vi "arduinoReadClock.vi"(8 "error in":errorcluster, 11 "Arduino Resource":T1={"VISA resource"="", "Board Type"=enum."Uno", "Connection Type"=enum."USB / Serial", "Bytes Per Packet (15)"=15}) -> (0 "error out":errorcluster, 2 "resulting string":string, 3 "Arduino Resource 2":T1={"VISA resource"="", "Board Type"=enum."Uno", "Connection Type"=enum."USB / Serial", "Bytes Per Packet (15)"=15})   [LabVIEW 2019]
uses:
  <vilib>/LabVIEW Interface for Arduino/Type Defs/Arduino Resource.ctl
  <vilib>/LabVIEW Interface for Arduino/Type Defs/Board Type.ctl
  <vilib>/LabVIEW Interface for Arduino/LabVIEW Interface for Arduino.lvlib
panel:
  out "output string":string
  out "year":u8
  out "month":u8
  out "day":u8
  out "hours":u8
  out "minutes":u8
  out "seconds":u8
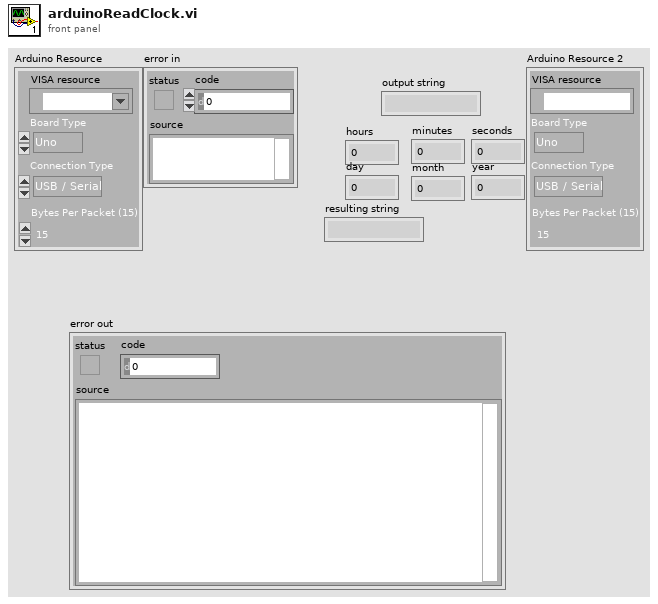
[diagram p1: front panel]
types:
  T1 = typedef "LabVIEW Interface for Arduino.lvlib/Arduino Resource.ctl" = cluster{"VISA resource":refnum<visa-resource-name>, "Board Type":T2, "Connection Type":enum8{"USB / Serial"}, "Bytes Per Packet (15)":u8}
  T2 = typedef "LabVIEW Interface for Arduino.lvlib/Board Type.ctl" = enum16{"Uno", "Dimuelanove w/Atmega 328", "Mega 2560"}
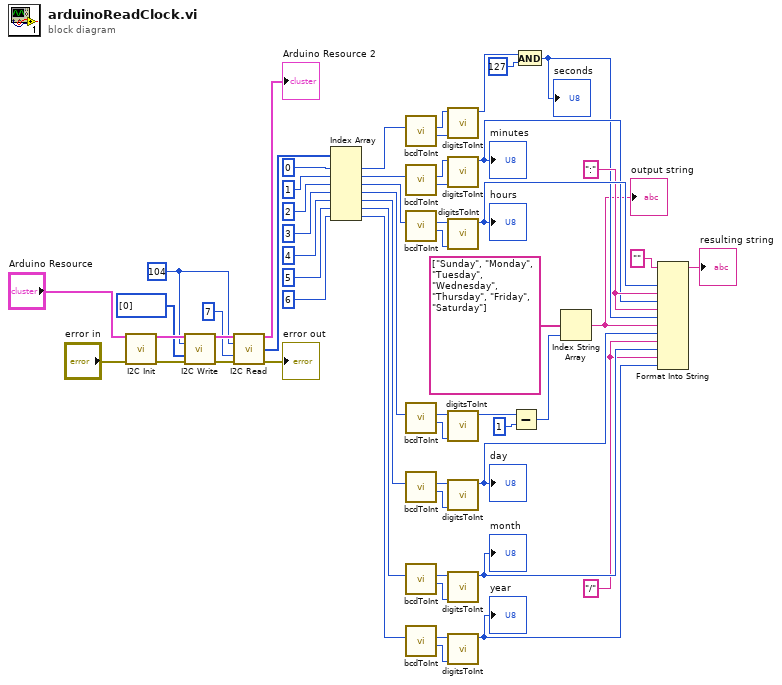
[diagram p0: block diagram]
diagram:
  w1 = "/"
  w7 = ":"
  w20 = u8 104 ("Address (0)")
  n1 = call <vilib>:"I2C Init.vi"("Arduino Resource"="Arduino Resource", "error in"="error in") -> ("Arduino Resource"=w57:T1, "error out"=w56:errorcluster)  [unwired: 12 in]
  n2 = call <vilib>:"I2C Write.vi"("Arduino Resource"=w57, "Address (0)"=w20, "I2C Data Bytes"=u8[] [0], "error in"=w56) -> ("Arduino Resource"=w54:T1, "error out"=w53:errorcluster)  [unwired: 10 in]
  n3 = call <vilib>:"I2C Read.vi"("Arduino Resource"=w54, "Address (0)"=w20, "Bytes To Read"=u8 7, "error in"=w53) -> ("Arduino Resource"=→"Arduino Resource 2":T1, "I2C Data"=w51:u8[], "error out"=→"error out":errorcluster)  [unwired: 9 in]
  n4 = Index Array(array=w51, index #1=0 ("index"), index #2=1 ("index"), index #3=2 ("index"), index #4=3 ("index"), index #5=4 ("index"), index #6=5 ("index"), index #7=6 ("index")) -> (element #1=w43:u8, element #2=w42:u8, element #3=w41:u8, element #4=w23:u8, element #5=w40:u8, element #6=w39:u8, element #7=w38:u8)
  n5 = call "bcdToInt.vi"("y"=w43) -> ("x .and. y?"=w36:u8, "x << y"=w37:u8)  [unwired: 9 in]
  n6 = call "bcdToInt.vi"("y"=w42) -> ("x .and. y?"=w27:u8, "x << y"=w26:u8)  [unwired: 9 in]
  n7 = call "bcdToInt.vi"("y"=w41) -> ("x .and. y?"=w29:u8, "x << y"=w28:u8)  [unwired: 9 in]
  n8 = call "bcdToInt.vi"("y"=w23) -> ("x .and. y?"=w25:u8, "x << y"=w24:u8)  [unwired: 9 in]
  n9 = call "bcdToInt.vi"("y"=w40) -> ("x .and. y?"=w31:u8, "x << y"=w30:u8)  [unwired: 9 in]
  n10 = call "bcdToInt.vi"("y"=w39) -> ("x .and. y?"=w33:u8, "x << y"=w32:u8)  [unwired: 9 in]
  n11 = call "bcdToInt.vi"("y"=w38) -> ("x .and. y?"=w34:u8, "x << y"=w35:u8)  [unwired: 9 in]
  n12 = call "digitsToInt.vi"("Numeric"=w36, "Numeric 2"=w37) -> ("x+y"=w22:u8)  [unwired: 9 in]
  n13 = call "digitsToInt.vi"("Numeric"=w27, "Numeric 2"=w26) -> ("x+y"=w6:u8)  [unwired: 9 in]
  "minutes" <- w6
  n14 = call "digitsToInt.vi"("Numeric"=w29, "Numeric 2"=w28) -> ("x+y"=w8:u8)  [unwired: 9 in]
  "hours" <- w8
  n15 = call "digitsToInt.vi"("Numeric"=w25, "Numeric 2"=w24) -> ("x+y"=w17:u8)  [unwired: 9 in]
  n16 = call "digitsToInt.vi"("Numeric"=w31, "Numeric 2"=w30) -> ("x+y"=w3:u8)  [unwired: 9 in]
  "day" <- w3
  n17 = call "digitsToInt.vi"("Numeric"=w33, "Numeric 2"=w32) -> ("x+y"=w2:u8)  [unwired: 9 in]
  "month" <- w2
  n18 = call "digitsToInt.vi"("Numeric"=w34, "Numeric 2"=w35) -> ("x+y"=w9:u8)  [unwired: 9 in]
  "year" <- w9
  n19 = Subtract(x=w17, y=u8 1) -> (x-y=w16:u8)
  n20 = And(x=w22, y=u8 127) -> (x .and. y?=w5:u8)
  "seconds" <- w5
  n21 = Index String Array(1:w16, 2:string[] ["Sunday", "Monday", "Tuesday", "Wednesday", "Thursday", "Friday", "Saturday"] ("string array")) -> (0:w4:string)  [unwired: 1 in]
  "output string" <- w4
  n22 = Format Into String(initial string="", w8, w7, w6, w7, w5, w4, w3, w1, w2, w1, w9) -> (resulting string=→"resulting string":string)  [unwired: 2 in, 1 out]
